vi "Measure and FPGA Align.vi"(0 "Register Buses":T1[](array[typedef]), 11 "error in":errorcluster, 12 "sync.cptr.period":u16[](array[numeric])) -> (4 "Register Buses (out)":T1[](array[typedef]), 15 "error out":errorcluster)   [LabVIEW 2014, in "ni579x Synchronization v2 Host.lvlib"]
uses:
  <instrlib>/ni579x/Synchronization/v2/Host/ni579x Synchronization v2 Host.lvlib
  <instrlib>/_niInstr/Register Bus/v0/Host/Public/Register Bus Session.ctl
  <instrlib>/_niInstr/Register Bus/v0/Host/Private/Session Data.ctl
  <vilib>/ErrorRing/Error Ring.xnode
  <instrlib>/_niInstr/Register Bus/v0/Host/niInstr Register Bus v0 Host.lvlib
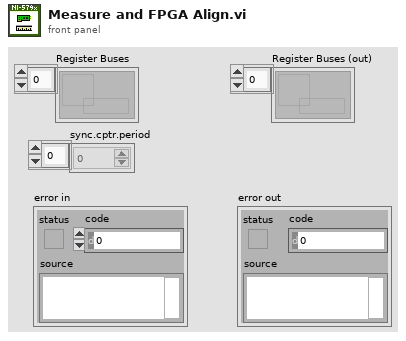
[diagram p1: front panel]
types:
  T1 = typedef "niInstr Register Bus v0 Host.lvlib/Register Bus Session.ctl" = refnum<queue>
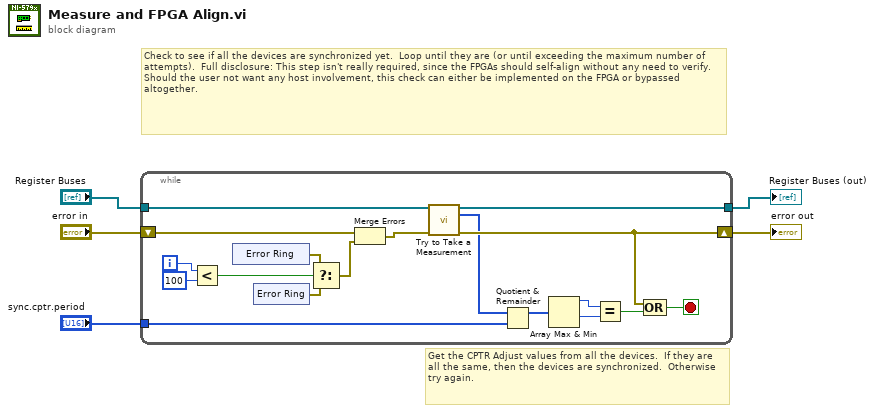
[diagram p0: block diagram]
diagram:
  # "Get the CPTR Adjust values from all the devices.  If they are all the same, then the devices are synchronized.  Otherwise try again."
  # "Check to see if all the devices are synchronized yet.  Loop until they are (or until exceeding the maximum number of attempts).  Full disclosure: This step isn't really required, since the FPGAs should self-align without any need to verify.  Should the user not want any host involvement, this check can either be implemented on the FPGA or bypassed altogether."
  n1 = while {
    tunnel: "sync.cptr.period" -> [w12]
    shift-right: [w16] -> w4
    shift-left: "error in" -> [w18]
    tunnel: "Register Buses" -> [w7]
    tunnel: [w6] -> w1
    i -> [w20]
    stop <- w21 stop-if-true
    n2 = Less?(x=w20, y=100 ("x")) -> (x < y?=w9:bool)
    n3 = xnode ("Error Ring")() -> ("error out"=w10:errorcluster)
    n4 = xnode ("Error Ring")() -> ("error out"=w11:errorcluster)
    n5 = Select(t=w10, s=w9, f=w11) -> (s? t:f=w8:errorcluster)
    n6 = Merge Errors(w18, w8) -> (w15:errorcluster)
    n7 = call <instrlib>:"Try to Take a Measurement.vi"("Register Buses"=w7, "error in"=w15) -> ("Register Buses (out)"=w6:T1[], "measurement values"=w14:u16[], "error out"=w16:errorcluster)  [unwired: 11 in]
    n8 = Quotient & Remainder(x=w14, y=w12) -> (x-y*floor(x/y)=w13:u16[])  [unwired: 1 out]
    n9 = Array Max & Min(array=w13) -> (max value=w23:u16, min value=w22:u16)  [unwired: 2 out]
    n10 = Equal?(x=w23, y=w22) -> (x = y?=w17:bool)
    n11 = Compound Arithmetic op=OR(w16, w17) -> (w21:bool)
  }
  "error out" <- w4
  "Register Buses (out)" <- w1
